vi "APC_9056_LoadINI.vi"   [LabVIEW 2020]
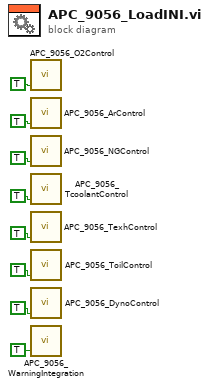
[diagram p0: block diagram]
diagram:
  n1 = call "APC_9056_O2Control.vi"("LoadIni?"=TRUE) -> ()  [unwired: 2 in, 1 out]
  n2 = call "APC_9056_ArControl.vi"("LoadIni?"=TRUE) -> ()  [unwired: 2 in, 1 out]
  n3 = call "APC_9056_NGControl.vi"("LoadIni?"=TRUE) -> ()  [unwired: 2 in, 1 out]
  n4 = call "APC_9056_TcoolantControl.vi"("LoadIni?"=TRUE) -> ()  [unwired: 2 in, 1 out]
  n5 = call "APC_9056_TexhControl.vi"("LoadIni?"=TRUE) -> ()  [unwired: 2 in, 1 out]
  n6 = call "APC_9056_ToilControl.vi"("LoadIni?"=TRUE) -> ()  [unwired: 2 in, 1 out]
  n7 = call "APC_9056_DynoControl.vi"("LoadIni?"=TRUE) -> ()  [unwired: 2 in, 1 out]
  n8 = call "APC_9056_WarningIntegration.vi"("LoadIni?"=TRUE) -> ()  [unwired: 7 in, 1 out]
